vi "UI_result.vi"(7 "result":T1=enum."OK", 8 "error in (no error)":errorcluster) -> (0 "error out":errorcluster)   [LabVIEW 2019]
uses:
  result.ctl
  _ctrl/rw.ctl
  SubVIs/common/Glob_setting.vi
  Global 1.vi
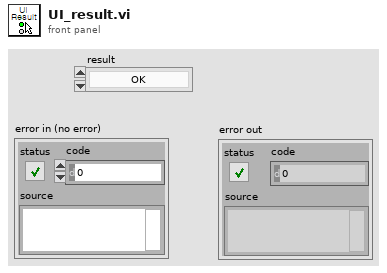
[diagram p1: front panel]
types:
  T1 = typedef "result.ctl" = enum16{"Init", "OK", "NG", "Shutdown", "Testing", "Completion", "Device Error", "Start", "작동", "미작동", "작동 대기", "작동 1"}
  T2 = typedef "rw.ctl" = enum16{"read", "write"}
  T3 = typedef "cap_config.ctl" = cluster{"Test Mode":enum32{"6.3.2 저온 작동/방치 시험", "6.3.3 고온 작동/방치 시험", "6.3.4 온도 싸이클 시험", "6.3.6 온습도 싸이클 시험", "6.3.8 결로 시험", "6.3.9 빙결 시험"}, "ON time[ms]":dbl, "OFF time[ms]":dbl, "1. 작동시간[분]":dbl, "2. 미작동시간[분]":dbl, "3. 작동시간[분]":dbl, "level[V]":dbl, "duty":dbl, "Freq":dbl, "Voltage+[V]":dbl, "Voltage-[V]":dbl, "Current+[A]":dbl, "Current-[A]":dbl, "출력전압[V]":dbl, "출력전류[A]":dbl, "OVP Level":dbl, "OCP Level":dbl, "Time Div":u16, "Record Len":i32, "방전 기준[V]":dbl, "Repeate (Each Ch)":u32, "Cycle[N]":u32, "ON/OFF 회 수[N]":dbl, "TrigPos[%]":dbl, "시험시간[분]":dbl}
  T4 = enum32{"6.3.2 저온 작동/방치 시험", "6.3.3 고온 작동/방치 시험", "6.3.4 온도 싸이클 시험", "6.3.6 온습도 싸이클 시험", "6.3.8 결로 시험", "6.3.9 빙결 시험"}
  T5 = typedef "Testing-info.ctl" = cluster{"전체채널수":u8, "현재채널번호":u8, "Irms":dbl, "입력전압":dbl, "입력전류":dbl, "출력전압":dbl, "출력전류":dbl, "온도":dbl, "제어단 단선":bool, "제어단 단락":bool, "제어단 특성변화":bool, "출력단 단선":bool, "출력단 단락":bool, "출력단 특성변화":bool, "출력단 전압":bool, "카운트 일치":bool, "Irms 판정":bool, "온도":bool, "테스트 회수":u32, "TestType":T6, "현재회수":u32, "Ch selection":cluster{"1ch":bool, "2ch":bool, "3ch":bool, "4ch":bool, "5ch":bool, "6ch":bool}, "반복":u32, "Path":path, "파일생성주기":u32, "start time":dbl, "stop time":dbl, "현재반복회수":u32, "NG":cluster{"입출력 카운트":bool, "출력전류RMS":bool}}
  T6 = typedef "sequence_single.ctl" = enum16{"Register", "RC", "B1", "B2", "B3", "Oper_LV", "Oper_HV", "ContR_LV"}
  T7 = typedef "ui_dev-operator.ctl" = cluster{"Operation stutus":refnum<vi>, "Test Status":refnum<vi>, "Setting":refnum<vi>, "Manual":refnum<vi>, "Main":refnum<vi>, "RCstart":refnum<vi>, "채널선택":refnum<vi>, "시험명":refnum<vi>, "Tab Control_manual":refnum<vi>, "시험 모드":refnum<vi>, "HW check":refnum<vi>, "login":refnum<vi>, "logout":refnum<vi>}
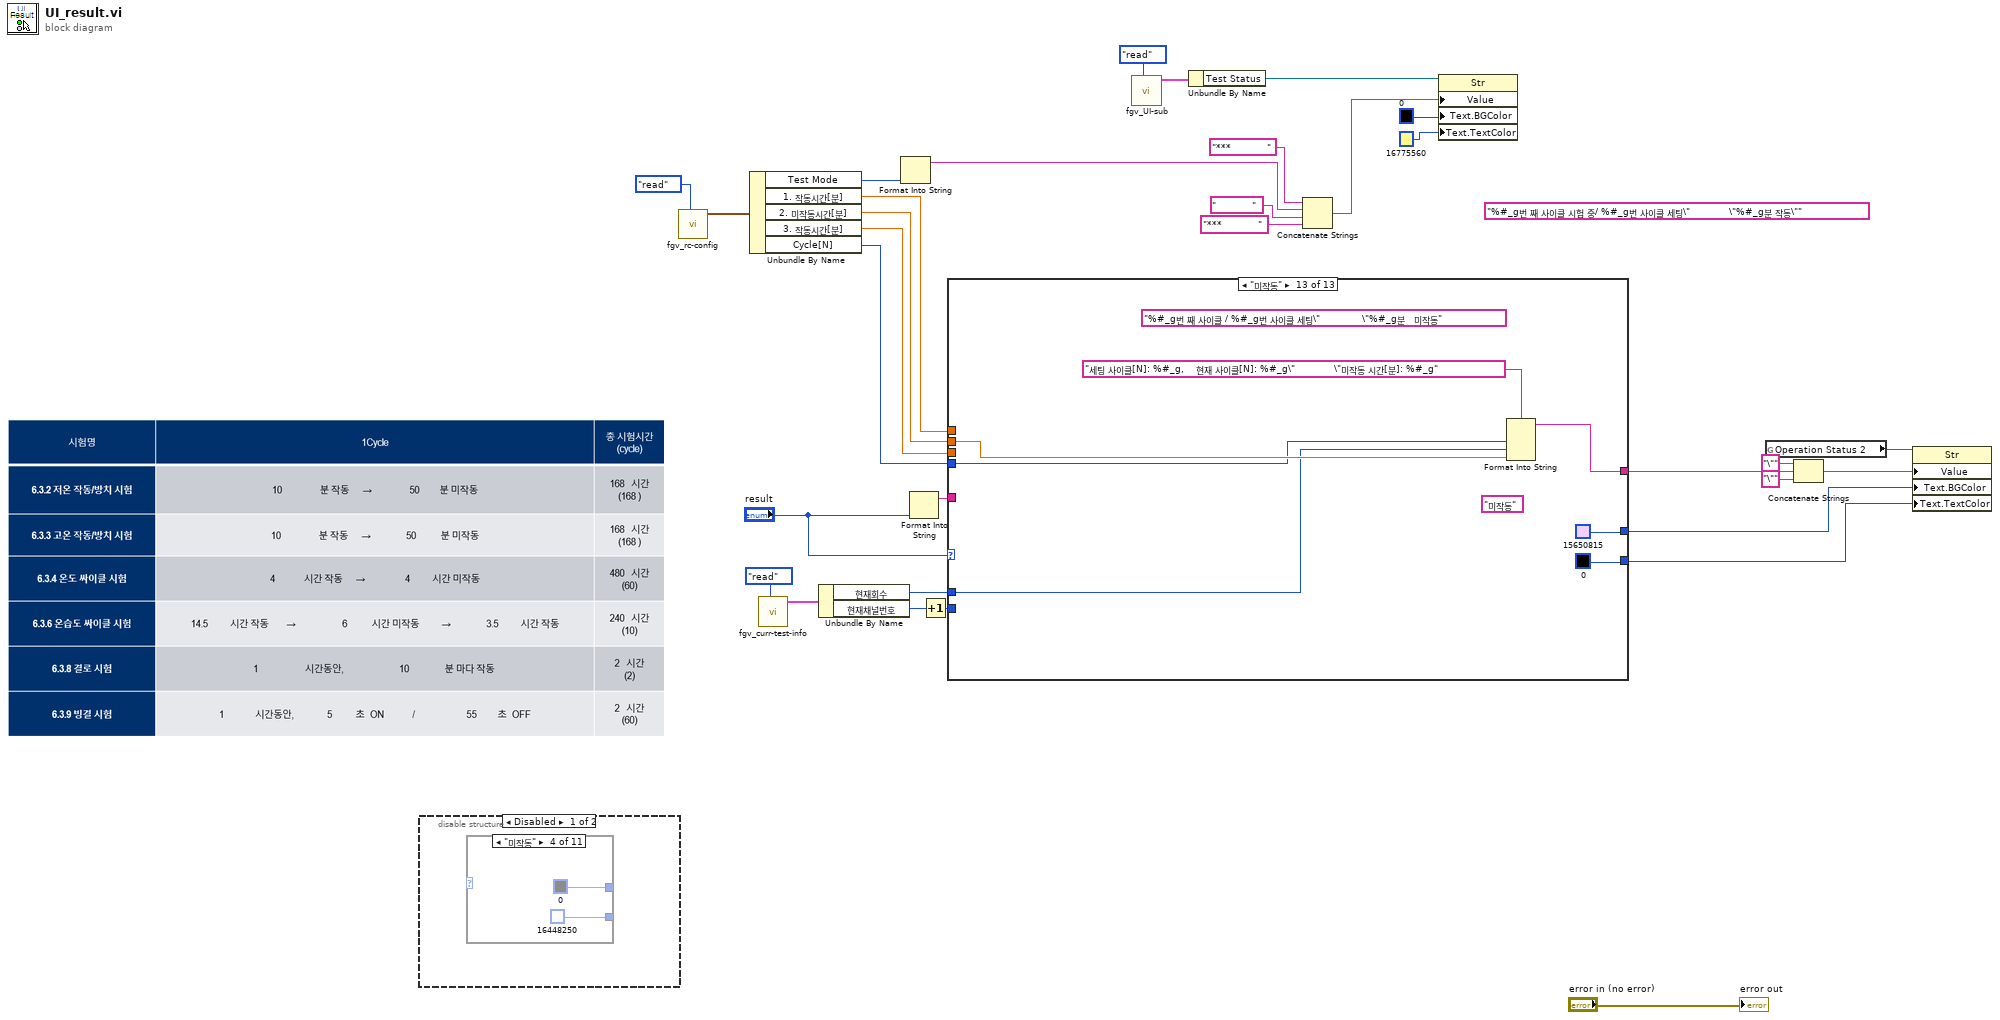
[diagram p0: block diagram]
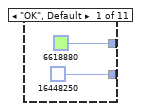
[diagram p2: hidden frame]
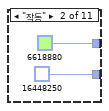
[diagram p3: hidden frame]
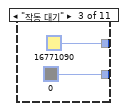
[diagram p4: hidden frame]
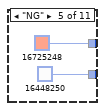
[diagram p5: hidden frame]
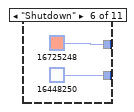
[diagram p6: hidden frame]
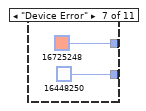
[diagram p7: hidden frame]
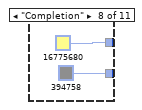
[diagram p8: hidden frame]
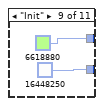
[diagram p9: hidden frame]
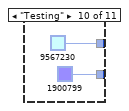
[diagram p10: hidden frame]
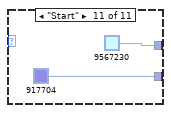
[diagram p11: hidden frame]
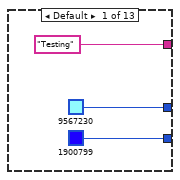
[diagram p13: hidden frame]
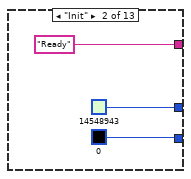
[diagram p14: hidden frame]
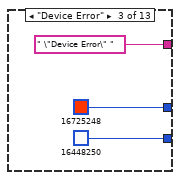
[diagram p15: hidden frame]
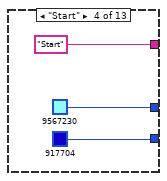
[diagram p16: hidden frame]
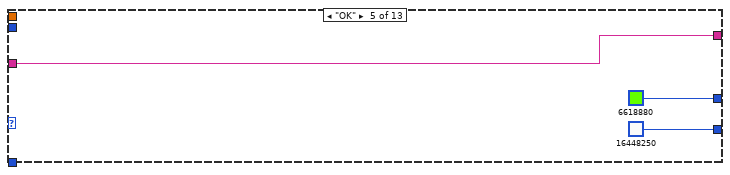
[diagram p17: hidden frame]
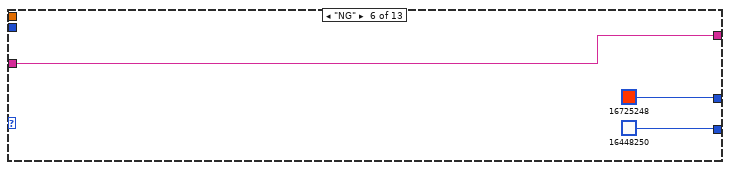
[diagram p18: hidden frame]
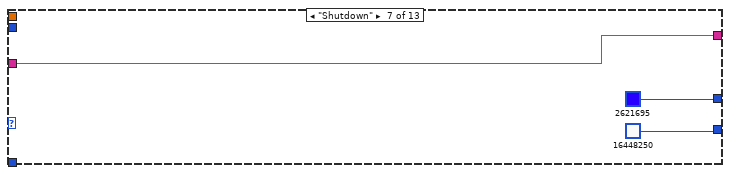
[diagram p19: hidden frame]
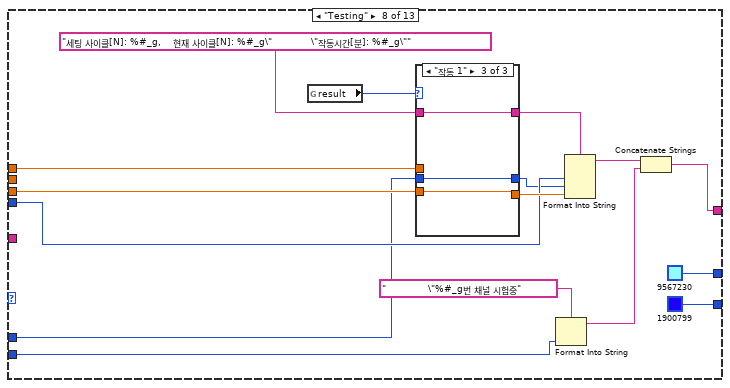
[diagram p20: hidden frame]
diagram:
  (unwired) "%#_g번 째 사이클 시험 중/ %#_g번 사이클 세팅\"             \"%#_g분 작동\"" ("Boolean Text.Text")
  n1 = disable-structure shown="Disabled" {
    frame Disabled {
      n2 = case shown="\"미작동\"" {
        selector: _ -> [_ _ _ _ _ _ _ _ _ _ _]
        tunnel: [u32 16448250 u32 16448250 u32 0 u32 16448250 u32 16448250 u32 16448250 u32 16448250 u32 394758 u32 16448250 u32 1900799 u32 917704] -> _
        tunnel: [u32 6618880 u32 6618880 u32 16771090 u32 0 u32 16725248 u32 16725248 u32 16725248 u32 16775680 u32 6618880 u32 9567230 u32 9567230] -> _
        frame "OK", Default {
        }
        frame "작동" {
        }
        frame "작동 대기" {
        }
        frame "미작동" {
        }
        frame "NG" {
        }
        frame "Shutdown" {
        }
        frame "Device Error" {
        }
        frame "Completion" {
        }
        frame "Init" {
        }
        frame "Testing" {
        }
        frame "Start" {
        }
      }
    }
    frame Enabled {
    }
  }
  n3 = call "fgv_rc-config.vi"("cmd"=rw."read") -> ("Testconfig out"=w25:T3)  [unwired: 9 in, 1 out]
  n4 = Unbundle By Name(w25) -> ("Test Mode"=w24:T4, "1. 작동시간[분]"=w19:dbl, "2. 미작동시간[분]"=w18:dbl, "3. 작동시간[분]"=w17:dbl, "Cycle[N]"=w1:u32)
  n5 = call "fgv_curr-test-info.vi"("cmd"=rw."read") -> ("현재테스트 정보 2"=w16:T5)  [unwired: 10 in]
  n6 = Unbundle By Name(w16) -> ("현재회수"=w14:u32, "현재채널번호"=w13:u8)
  n7 = Format Into String(w24) -> (resulting string=w21:string)  [unwired: 3 in, 1 out]
  n8 = Format Into String("result") -> (resulting string=w29:string)  [unwired: 3 in, 1 out]
  n9 = Increment(x=w13) -> (x+1=w12:u8)
  n10 = case shown="\"미작동\"" "result" {
    selector: "result" -> [_ _ _ _ _ _ _ _ w107 _ _ _ _]
    tunnel: ["Testing" "Ready" " \"Device Error\" " "Start" w69 w72 w75 w84 w104 w110 w116 w125 w131] -> w9
    tunnel: w29 -> [_ _ _ _ w69 w72 w75 _ _ _ _ _ _]
    tunnel: [u32 9567230 u32 14548943 u32 16725248 u32 9567230 u32 6618880 u32 16725248 u32 2621695 u32 9567230 u32 16775680 u32 6618880 u32 6618880 u32 9567230 u32 15650815] -> w5
    tunnel: [u32 1900799 u32 0 u32 16448250 u32 917704 u32 16448250 u32 16448250 u32 16448250 u32 1900799 u32 394758 u32 16448250 u32 16448250 u32 1900799 u32 0] -> w4
    tunnel: w19 -> [_ _ _ _ _ _ _ w87 _ w112 _ w124 _]
    tunnel: w18 -> [_ _ _ _ _ _ _ _ _ _ _ _ w130]
    tunnel: w17 -> [_ _ _ _ _ _ _ w79 _ _ w115 _ _]
    tunnel: w14 -> [_ _ _ _ _ _ _ w76 w101 _ _ w120 w127]
    tunnel: w12 -> [_ _ _ _ _ _ _ w82 _ _ _ _ _]
    tunnel: w1 -> [_ _ _ _ _ _ _ w78 w102 _ _ w121 w128]
    frame Default {
    }
    frame "Init" {
    }
    frame "Device Error" {
    }
    frame "Start" {
    }
    frame "OK" {
    }
    frame "NG" {
    }
    frame "Shutdown" {
    }
    frame "Testing" {
      n11 = global read "Glob_setting.vi" "result"() -> (w89:T1)
      n12 = case shown="\"작동 1\"" w89 {
        tunnel: "세팅 사이클[N]: %#_g,    현재 사이클[N]: %#_g\"             \"작동시간[분]: %#_g\"" ("Boolean Text.Text") -> [_ w97 w100]
        tunnel: w87 -> [_ w96 _]
        tunnel: ["" ("Boolean Text.Text") w97 w100] -> w86
        tunnel: [0.0 ("1. 작동시간[분]") w96 w98] -> w80
        tunnel: [u32 0 ("현재회수") w95 w99] -> w77
        tunnel: w76 -> [_ w95 w99]
        tunnel: w79 -> [_ _ w98]
        frame "Init", Default {
        }
        frame "작동" {
        }
        frame "작동 1" {
        }
      }
      n13 = Format Into String(format string="              \"%#_g번 채널 시험중" ("Boolean Text.Text"), w82) -> (resulting string=w81:string)  [unwired: 2 in, 1 out]
      n14 = Format Into String(format string=w86, w78, w77, w80) -> (resulting string=w85:string)  [unwired: 2 in, 1 out]
      n15 = Concatenate Strings(w85, w81) -> (w84:string)
    }
    frame "Completion" {
      (unwired) "%#_g번 째 사이클 / %#_g 사이클\"             " ("Boolean Text.Text")
      n16 = global write "Glob_setting.vi" "result"(w107) -> ()
      n17 = Format Into String(format string="세팅 사이클[N]: %#_g,    현재 사이클[N]: %#_g\"           " ("Boolean Text.Text"), w102, w101) -> (resulting string=w106:string)  [unwired: 2 in, 1 out]
      n18 = Concatenate Strings(w106, "\"시험 완료" ("Boolean Text.Text")) -> (w104:string)
    }
    frame "작동" {
      n19 = Format Into String(format string="%#_g분   작동" ("Boolean Text.Text"), w112) -> (resulting string=w110:string)  [unwired: 2 in, 1 out]
    }
    frame "작동 1" {
      n20 = Format Into String(format string="%#_g분   작동" ("Boolean Text.Text"), w115) -> (resulting string=w116:string)  [unwired: 2 in, 1 out]
    }
    frame "작동 대기" {
      (unwired) "세팅 사이클[N]: %#_g,    현재 사이클[N]: %#_g\"             \"미작동 시간[분]: %#_g\"" ("Boolean Text.Text")
      n21 = Format Into String(format string="세팅 사이클[N]: %#_g,    현재 사이클[N]: %#_g\"           \"%#_g분 작동대기" ("Boolean Text.Text"), w121, w120, w124) -> (resulting string=w125:string)  [unwired: 2 in, 1 out]
    }
    frame "미작동" {
      (unwired) "%#_g번 째 사이클 / %#_g번 사이클 세팅\"              \"%#_g분   미작동" ("Boolean Text.Text")
      (unwired) "미작동" ("Boolean Text.Text")
      n22 = Format Into String(format string="세팅 사이클[N]: %#_g,    현재 사이클[N]: %#_g\"             \"미작동 시간[분]: %#_g" ("Boolean Text.Text"), w128, w127, w130) -> (resulting string=w131:string)  [unwired: 2 in, 1 out]
    }
  }
  n23 = call "fgv_UI-sub.vi"("cmd"=rw."read") -> ("output cluster 2"=w31:T7)  [unwired: 9 in, 1 out]
  n24 = Unbundle By Name(w31) -> ("Test Status"=w32:refnum<vi>)
  n25 = Concatenate Strings("***            " ("string"), w21, "            " ("string"), "***            " ("string")) -> (w11:string)
  n26 = property class="Str"(reference=w32, "Value"=w11, "Text.BGColor"=u32 0, "Text.TextColor"=u32 16775560) -> ()  [unwired: 1 in, 2 out]
  n27 = global read "Global 1.vi" "Operation Status 2"() -> (w7:refnum<vi>)
  n28 = Concatenate Strings("\"" ("string"), w9, "\"" ("string")) -> (w6:string)
  n29 = property class="Str"(reference=w7, "Value"=w6, "Text.BGColor"=w5, "Text.TextColor"=w4) -> ()  [unwired: 1 in, 2 out]
  "error out" <- "error in (no error)"
